vi "Write.vi"(8 "error in (no error)":errorcluster, 9 "Parameter 2":string="1", 10 "Parameter 1":string="DI", 11 "LifterTCP in":refnum<class "LifterTCP.lvclass">) -> (0 "error out":errorcluster, 2 "Driver ACK?":bool, 3 "LifterTCP out":refnum<class "LifterTCP.lvclass">)   [LabVIEW 2019, in "LifterTCP.lvclass"]
uses:
  LifterTCP.lvclass
  LifterTCP.lvclass/LifterTCP.ctl
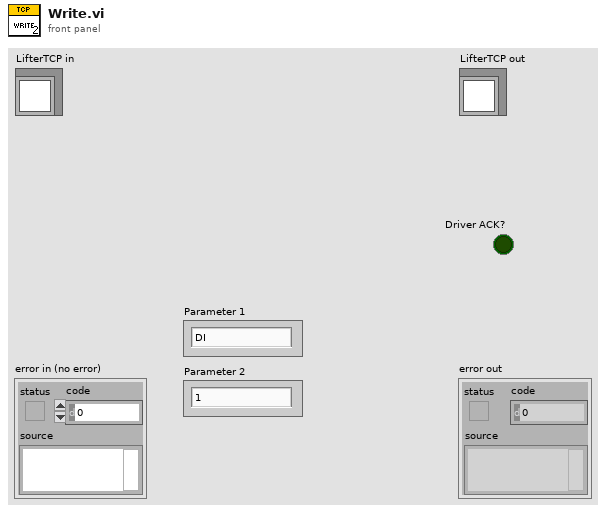
[diagram p1: front panel]
types:
  T1 = typedef "Semaphore RefNum" = refnum<k1>
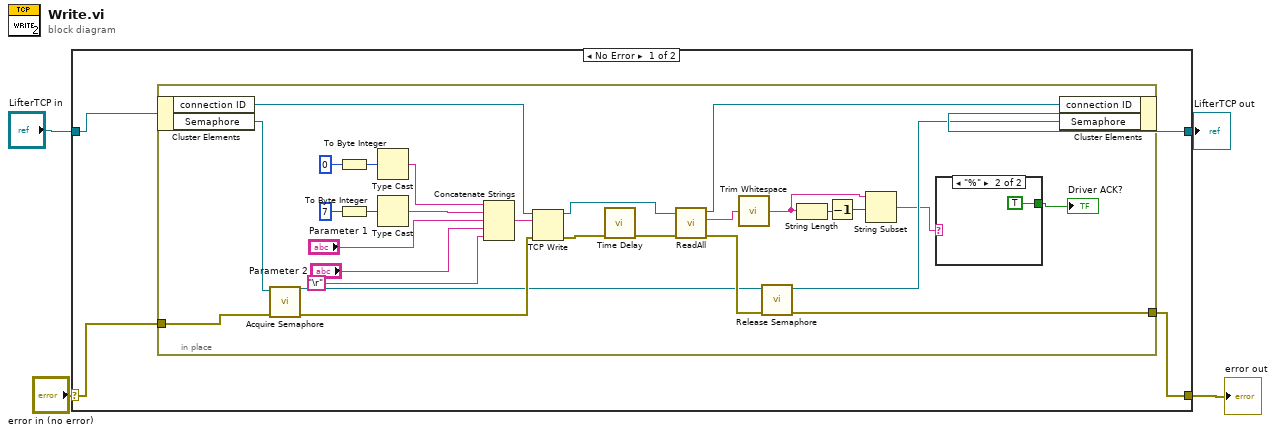
[diagram p0: block diagram]
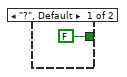
[diagram p2: hidden frame]
diagram:
  n1 = case shown="No Error" "error in (no error)" {
    selector: "error in (no error)" -> [w8 w40]
    tunnel: [w7 w40] -> w3
    tunnel: [w6 w39] -> w1
    tunnel: "LifterTCP in" -> [w5 w39]
    frame No Error {
      n2 = in-place {
        in-place-border: w8 -> [w26]
        in-place-border: [w18] -> w7
        n3 = in-place-cluster #1(w5) -> ("connection ID"=w17:refnum<k5>, "Semaphore"=w27:T1)
        n4 = call <vilib>:"Acquire Semaphore.vi"("error in (no error)"=w26, "semaphore"=w27) -> ("error out"=w25:errorcluster, "semaphore out"=w20:T1)  [unwired: 3 in, 1 out]
        n5 = To Byte Integer(number=i8 0) -> (8bit integer=w33:i8)
        n6 = To Byte Integer(number=i8 7) -> (8bit integer=w36:i8)
        n7 = Type Cast(x=w33) -> (*(type *) &x=w34:string)  [unwired: 1 in]
        n8 = Type Cast(x=w36) -> (*(type *) &x=w35:string)  [unwired: 1 in]
        n9 = Concatenate Strings(w34, w35, "Parameter 1", "Parameter 2", "\r") -> (w28:string)
        n10 = TCP Write(connection ID=w17, data in=w28, error in (no error)=w25) -> (connection ID out=w21:refnum<k5>, error out=w29:errorcluster)  [unwired: 1 in, 1 out]
        n11 = call "Time Delay"("error in (no error)"=w29) -> ("error out"=w23:errorcluster)  [unwired: 10 in]
        n12 = call "ReadAll.vi"("error in (no error)"=w23, "connection ID"=w21) -> ("error out"=w22:errorcluster, "Read Data"=w13:string, "connection ID out"=w19:refnum<k5>)  [unwired: 7 in]
        n13 = call <vilib>:"Trim Whitespace.vi"("string"=w13) -> ("trimmed string"=w14:string)  [unwired: 1 in]
        n14 = call <vilib>:"Release Semaphore.vi"("error in (no error)"=w22, "semaphore"=w20) -> ("error out"=w18:errorcluster, "semaphore out"=w24:T1)  [unwired: 4 in]
        n15 = String Length(string=w14) -> (length=w16:i32)
        n16 = Decrement(x=w16) -> (x-1=w15:i32)
        n17 = String Subset(string=w14, offset (0)=w15) -> (substring=w11:string)  [unwired: 1 in]
        n18 = case shown="\"%\"" w11 {
          tunnel: [FALSE ("Command Executed 2") TRUE ("Command Executed 2")] -> w12
          frame "?", Default {
          }
          frame "%" {
          }
        }
        "Driver ACK?" <- w12
        n19 = in-place-cluster #1("connection ID"=w19, "Semaphore"=w24) -> (w6:refnum<class "LifterTCP.lvclass">)
      }
    }
    frame Error {
    }
  }
  "error out" <- w3
  "LifterTCP out" <- w1
